vi "UpdateMbEng.vi"(8 "error in (no error)":errorcluster, 10 "modbus":refnum<class "Modbus Master.lvclass">, 11 "NeedleValve in":refnum<class "NeedleValve.lvclass">) -> (0 "error out":errorcluster, 3 "NeedleValve out":refnum<class "NeedleValve.lvclass">)   [LabVIEW 2019, in "NeedleValve.lvclass"]
uses:
  NeedleValve.lvclass
  <vilib>/NI/Modbus Library/API/Master/Modbus Master.lvclass
  NeedleValve.lvclass/NeedleValve.ctl
  modbus engine custom/MB_MODULE_class/MB_MODULE.lvclass/MB_MODULE.ctl
  modbus engine custom/MB_ENGINE_class/MB_ENGINE.lvclass
  D:/GIT H4000/H4000/src/modbus engine custom/MB_MODULE_class/MB_MODULE.lvclass
  modbus engine custom/MB_MODULE_class/MB_MODULE.lvclass
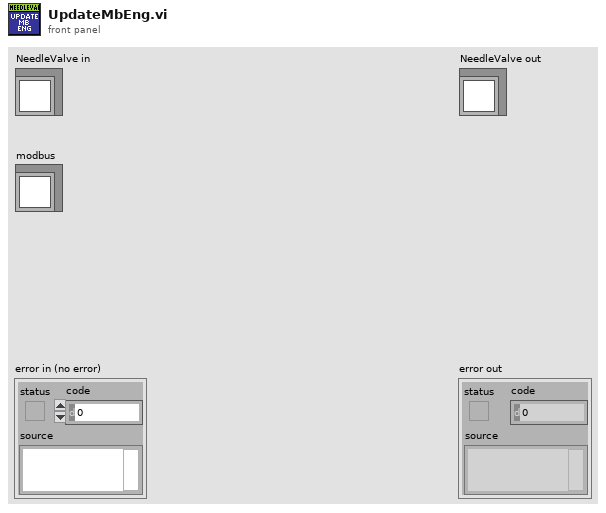
[diagram p1: front panel]
types:
  T1 = typedef "Needle Valve Data.ctl" = cluster{"Engine State":T2, "StateValveModbus":T3, "Alarms":T4, "RAW":i32, "Angele":dbl, "Step":i32, "Encoder":i32, "Kinematic":T5, "Limits":T6, "EncoderMax":i32, "Counter Max Dont Update":i32, "EncoderMin":i32, "Counter Min Dont Update":i32, "Prepere Counter":i32, "STEP INIT":i32, "offset - Angel":dbl}
  T2 = typedef "MB_ENGINE.lvclass/Engine State.ctl" = u16
  T3 = typedef "Needle Valve State.ctl" = enum16{"STOPED", "CLOSED", "OPENED", "OPENING", "CLOSING", "FULL_CLOSE", "PREP_OPEN"}
  T4 = typedef "MB_ENGINE.lvclass/Engine Alarms.ctl" = cluster{"OL":bool, "TF":bool, "STL":bool, "OCP":bool, "CPUV":bool, "UVLO":bool, "SPI_ERROR":bool, "Fault":bool, "OL 2":bool, "TF 2":bool, "STL 2":bool, "OCP 2":bool, "CPUV 2":bool, "UVLO 2":bool, "reserved":bool, "InitDone":bool}
  T5 = typedef "MB_ENGINE.lvclass/Settings.ctl" = cluster{"ACC Steps Per Sec^2":u16, "DEC Steps Per Sec^2":u16, "Min Velosity Step Per Sec":u16, "Max Velosity Step Per Sec":u16, "MicroStep":u16}
  T6 = typedef "MB_ENGINE.lvclass/Limits Status.ctl" = cluster{"Fault 2 Switch":bool, "Fault 1 Switch":bool, "Center(Home)":bool, "Lower Limit":bool, "Upper Limit":bool}
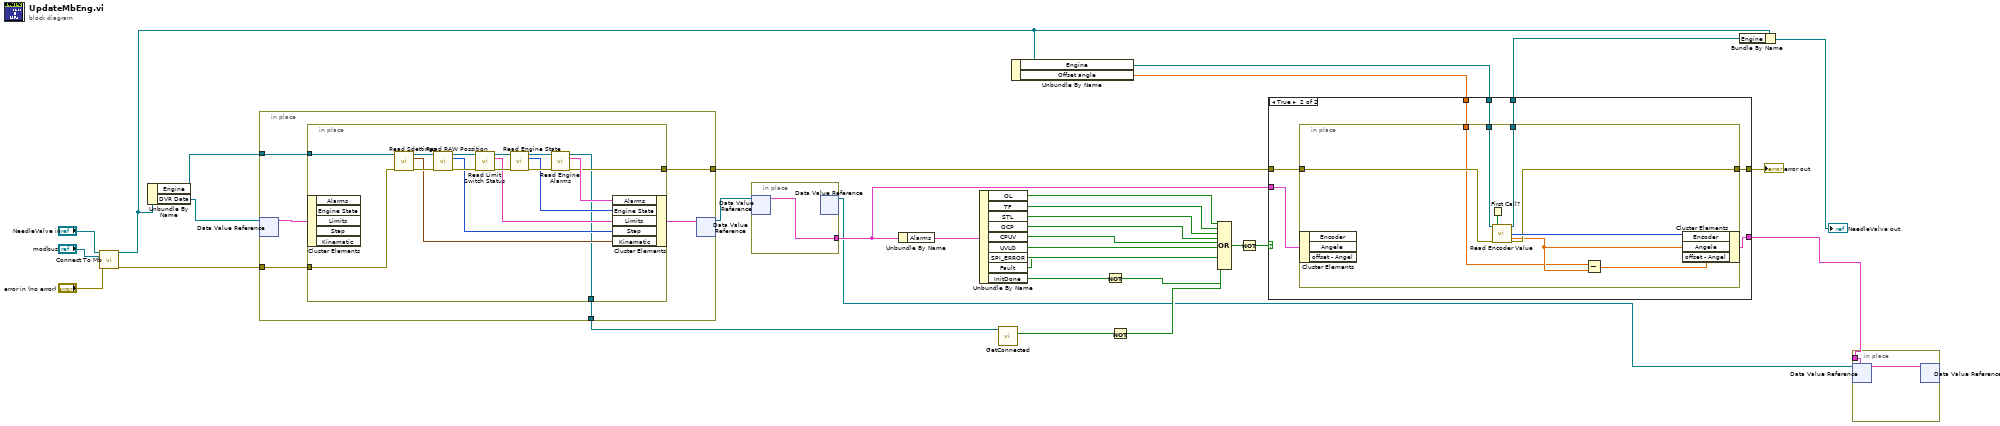
[diagram p0: block diagram]
diagram:
  n1 = call "Connect To Mb.vi"("reference in"="NeedleValve in", "modbus"="modbus", "error in (no error)"="error in (no error)") -> ("reference out"=w7:refnum<class "NeedleValve.lvclass">, "error out"=w19:errorcluster)  [unwired: 11 in]
  n2 = Unbundle By Name(w7) -> ("Engine"=w10:refnum<class "MB_ENGINE.lvclass">, "DVR Data"=w11:refnum<data-value>)
  n3 = in-place {
    in-place-border: [w39] -> w33
    in-place-border: w19 -> [w38]
    in-place-border: [w37] -> w17
    in-place-border: w10 -> [w35]
    n4 = in-place-dvr #1(w11) -> (w36:T1)  [unwired: 1 out]
    n5 = in-place {
      in-place-border: w38 -> [w43]
      in-place-border: [w42] -> w39
      in-place-border: [w41] -> w37
      in-place-border: w35 -> [w40]
      n6 = in-place-cluster #2(w36) -> ()  [unwired: 5 out]
      n7 = call "Read Sdettings.vi"("class data in"=w40, "error in (no error)"=w43) -> ("class data out"=w56:refnum<class "MB_ENGINE.lvclass">, "cluster"=w44:T5, "error out"=w52:errorcluster)  [unwired: 11 in]
      n8 = call "Read RAW Possition.vi"("class data in"=w56, "error in (no error)"=w52) -> ("class data out"=w55:refnum<class "MB_ENGINE.lvclass">, "RAW Possition"=w45:i32, "error out"=w51:errorcluster)  [unwired: 11 in]
      n9 = call "Read Limit Switch Status.vi"("class data in"=w55, "error in (no error)"=w51) -> ("class data out"=w54:refnum<class "MB_ENGINE.lvclass">, "Limits"=w46:T6, "error out"=w50:errorcluster)  [unwired: 11 in]
      n10 = call "Read Engine State.vi"("class data in"=w54, "error in (no error)"=w50) -> ("class data out"=w53:refnum<class "MB_ENGINE.lvclass">, "Engine State"=w47:T2, "error out"=w49:errorcluster)  [unwired: 11 in]
      n11 = call "Read Engine Alarms.vi"("class data in"=w53, "error in (no error)"=w49) -> ("class data out"=w41:refnum<class "MB_ENGINE.lvclass">, "Alarms"=w48:T4, "error out"=w42:errorcluster)  [unwired: 11 in]
      n12 = in-place-cluster #2("Alarms"=w48, "Engine State"=w47, "Limits"=w46, "Step"=w45, "Kinematic"=w44) -> (w34:T1)
    }
    n13 = in-place-dvr #1(w34) -> (w9:refnum<data-value>)  [unwired: 1 out]
  }
  n14 = in-place {
    in-place-border: [w57] -> w8
    n15 = in-place-dvr #3(w9) -> (w57:T1)  [unwired: 1 out]
    n16 = in-place-dvr #3() -> (w2:refnum<data-value>)  [unwired: 1 in, 1 out]
  }
  n17 = Unbundle By Name(w8) -> ("Alarms"=w12:T4)
  n18 = Unbundle By Name(w12) -> ("OL"=w31:bool, "TF"=w30:bool, "STL"=w29:bool, "OCP"=w28:bool, "CPUV"=w27:bool, "UVLO"=w26:bool, "SPI_ERROR"=w25:bool, "Fault"=w24:bool, "InitDone"=w15:bool)
  n19 = call "GetConnected.vi"("MB_MODULE in"=w17) -> ("Connected"=w16:bool)  [unwired: 10 in]
  n20 = Unbundle By Name(w7) -> ("Engine"=w6:refnum<class "MB_ENGINE.lvclass">, "Offset angle"=w3:dbl)
  n21 = Not(x=w15) -> (.not. x?=w14:bool)
  n22 = Not(x=w16) -> (.not. x?=w18:bool)
  n23 = Compound Arithmetic op=OR(w31, w30, w29, w28, w27, w26, w25, w24, w14, w18) -> (w23:bool)
  n24 = Not(x=w23) -> (.not. x?=w22:bool)
  n25 = case shown="True" w22 {
    tunnel: w8 -> [w59 w67]
    tunnel: [w59 w66] -> w1
    tunnel: w33 -> [w60 w65]
    tunnel: [w60 w64] -> w32
    tunnel: w6 -> [w58 w63]
    tunnel: [w58 w62] -> w5
    tunnel: w3 -> [_ w61]
    frame False {
    }
    frame True {
      n26 = in-place {
        in-place-border: [w73] -> w64
        in-place-border: w65 -> [w74]
        in-place-border: w63 -> [w70]
        in-place-border: [w69] -> w62
        in-place-border: w61 -> [w68]
        n27 = in-place-cluster #4(w67) -> ()  [unwired: 3 out]
        n28 = First Call?() -> (First Call?: T/F=w75:bool)
        n29 = call "Read Encoder Value.vi"("class data in"=w70, "init"=w75, "error in (no error)"=w74) -> ("class data out"=w69:refnum<class "MB_ENGINE.lvclass">, "Encoder"=w76:i32, "Angel (rad)"=w72:dbl, "error out"=w73:errorcluster)  [unwired: 8 in, 1 out]
        n30 = Subtract(x=w68, y=w72) -> (x-y=w71:dbl)
        n31 = in-place-cluster #4("Encoder"=w76, "Angele"=w72, "offset - Angel"=w71) -> (w66:T1)
      }
    }
  }
  "error out" <- w32
  n32 = Bundle By Name(cluster=w7, "Engine"=w5) -> (→"NeedleValve out":refnum<class "NeedleValve.lvclass">)
  n33 = in-place {
    in-place-border: w1 -> [w77]
    n34 = in-place-dvr #5(w2) -> ()  [unwired: 2 out]
    n35 = in-place-dvr #5(w77) -> ()  [unwired: 2 out]
  }
